vi "Configure Angle Limits.vi"(6 "Counter-Clockwise Angle Limit (300 deg)":dbl=300.0, 8 "error in (no error)":errorcluster, 9 "Clockwise Angle Limit (0 deg)":dbl, 10 "Motor ID (0)":u8, 11 "Dynamixel Motor VISA in":refnum<class "Dynamixel Motor VISA.lvclass">) -> (0 "error out":errorcluster, 3 "Dynamixel Motor VISA out":refnum<class "Dynamixel Motor VISA.lvclass">)   [LabVIEW 2016, in "Dynamixel Motor VISA.lvclass"]
doc: "This VI changes the angle limits of a motor."
uses:
  <instrlib>/Dynamixel Motor/HAIOL/VISA/Dynamixel Motor VISA.lvclass
  <instrlib>/Dynamixel Motor/HAIOL/VISA/Dynamixel Motor VISA.lvclass/Dynamixel Motor VISA.ctl
  <instrlib>/Dynamixel Motor/Dynamixel Motor.lvlib
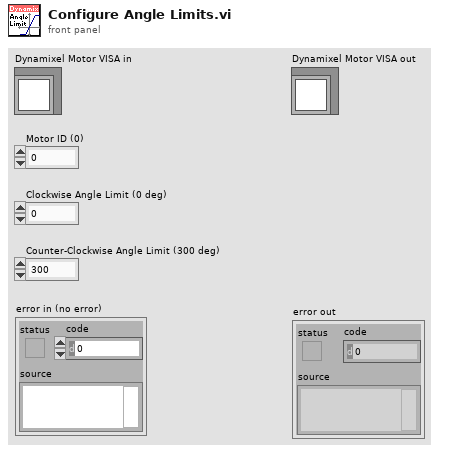
[diagram p1: front panel]
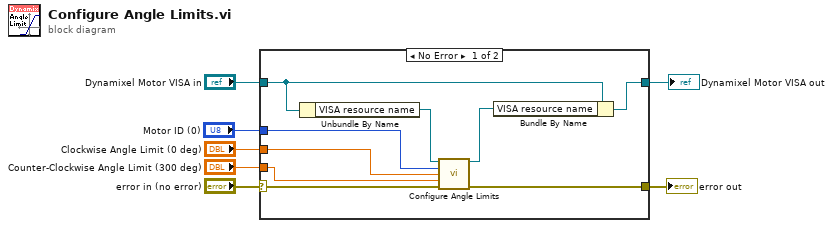
[diagram p0: block diagram]
diagram:
  n1 = case shown="No Error" "error in (no error)" {
    selector: "error in (no error)" -> [w16 w17]
    tunnel: "Dynamixel Motor VISA in" -> [w9 w18]
    tunnel: "Motor ID (0)" -> [w14 _]
    tunnel: "Clockwise Angle Limit (0 deg)" -> [w13 _]
    tunnel: "Counter-Clockwise Angle Limit (300 deg)" -> [w12 _]
    tunnel: [w11 w17] -> w2
    tunnel: [w8 w18] -> w1
    frame No Error {
      n2 = Unbundle By Name(w9) -> ("VISA resource name"=w15:refnum<visa-resource-name>)
      n3 = call <instrlib>:"Configure Angle Limits.vi"("VISA resource name"=w15, "Motor ID (0)"=w14, "Clockwise Angle Limit (0 deg)"=w13, "Counter-Clockwise Angle Limit (300 deg)"=w12, "error in (no error)"=w16) -> ("VISA resource name out"=w10:refnum<visa-resource-name>, "error out"=w11:errorcluster)  [unwired: 9 in]
      n4 = Bundle By Name(cluster=w9, "VISA resource name"=w10) -> (w8:refnum<class "Dynamixel Motor VISA.lvclass">)
    }
    frame Error {
    }
  }
  "error out" <- w2
  "Dynamixel Motor VISA out" <- w1
